vi "Configure Setpoint Number.vi"(8 "error in (no error)":errorcluster, 9 "Setpoint Number (0)":i16 min=0 max=17, 11 "VISA resource name":refnum<visa-resource-name>) -> (0 "error out":errorcluster, 3 "VISA resource name out":refnum<visa-resource-name>)   [LabVIEW 2012, in "Temptronic TP04300.lvlib"]
doc: "This VI configures setpoint number.\n\n<b>Setpoint Number</b> configures setpoint number\nDefault Value: 0\nValid range: 0 - 17 - for the Cycle Screen\n 0 - 2 - for the Operator Screen"
uses:
  <instrlib>/Temptronic TP04300/Temptronic TP04300.lvlib
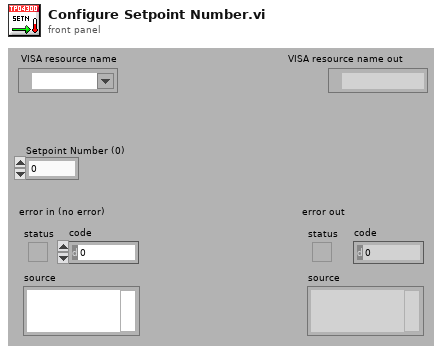
[diagram p1: front panel]
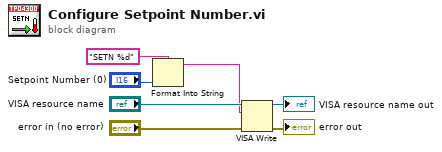
[diagram p0: block diagram]
diagram:
  n1 = Format Into String(format string="SETN %d" ("multi-line string"), "Setpoint Number (0)") -> (resulting string=w3:string)  [unwired: 2 in, 1 out]
  n2 = VISA Write(VISA resource name="VISA resource name", write buffer=w3, error in (no error)="error in (no error)") -> (VISA resource name out=→"VISA resource name out":refnum<visa-resource-name>, error out=→"error out":errorcluster)  [unwired: 1 out]
